vi "BalloonChannelControl.vi"(8 "error in":errorcluster) -> (0 "error out":errorcluster, 3 "task out":refnum<k21>)   [LabVIEW 2018]
uses:
  <vilib>/DAQmx/create/channels.llb/DAQmx Create Channel (DO-Digital Output).vi
  <resource>/objmgr/daqmx.rc
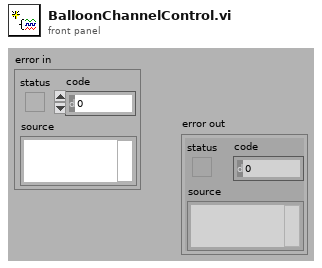
[diagram p1: front panel]
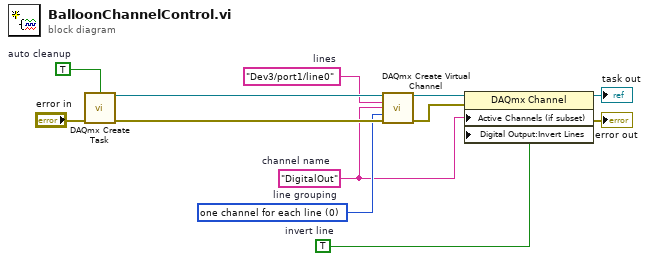
[diagram p0: block diagram]
diagram:
  w2 = TRUE  # invert line
  w7 = 0 items=["one channel for each line", "one channel for all lines"]  # line grouping
  w1 = "DigitalOut"  # channel name
  w8 = "Dev3/port1/line0"  # lines
  w10 = TRUE  # auto cleanup
  n1 = call <vilib>:"DAQmx Create Task.vi"("auto cleanup"=w10, "error in"="error in") -> ("task out"=w9:refnum<k21>, "error out"=w11:errorcluster)  [unwired: 12 in]
  n2 = call-poly <vilib>:"DAQmx Create Virtual Channel.vi"("task in"=w9, "lines"=w8, "name to assign"=w1, "line grouping"=w7, "error in"=w11) -> ("task out"=w6:refnum<k21>, "error out"=w5:errorcluster)  [unwired: 9 in]
  n3 = property class="DAQmx Channel"(reference=w6, error in=w5, "Active Channels (if subset)"=w1, "Digital Output:Invert Lines"=w2) -> (reference out=→"task out":refnum<k21>, error out=→"error out":errorcluster)
